vi "Draw Icon.vi"(6 "State":T2, 7 "Sizes":T1, 11 "Picture  In":picture) -> (3 "Picture":picture)   [LabVIEW 2020, in "FlexBlock.xnode"]
uses:
  FlexBlock.xnode
  State.ctl
  FlexBlocks/Type Descriptor.ctl
  FlexBlocks/Terminal Direction.ctl
  FlexBlocks/Value Mode.ctl
  FlexBlocks/Terminal State.ctl
  FlexBlocks/Special Terminal.ctl
  FlexBlocks/Errors.ctl
  <vilib>/picture/picture.llb/imagedata.ctl
  FlexBlocks/Calculated Sizes.ctl
  FlexBlocks/Size Constants.ctl
  FlexBlocks/FlexBlocks.lvlib
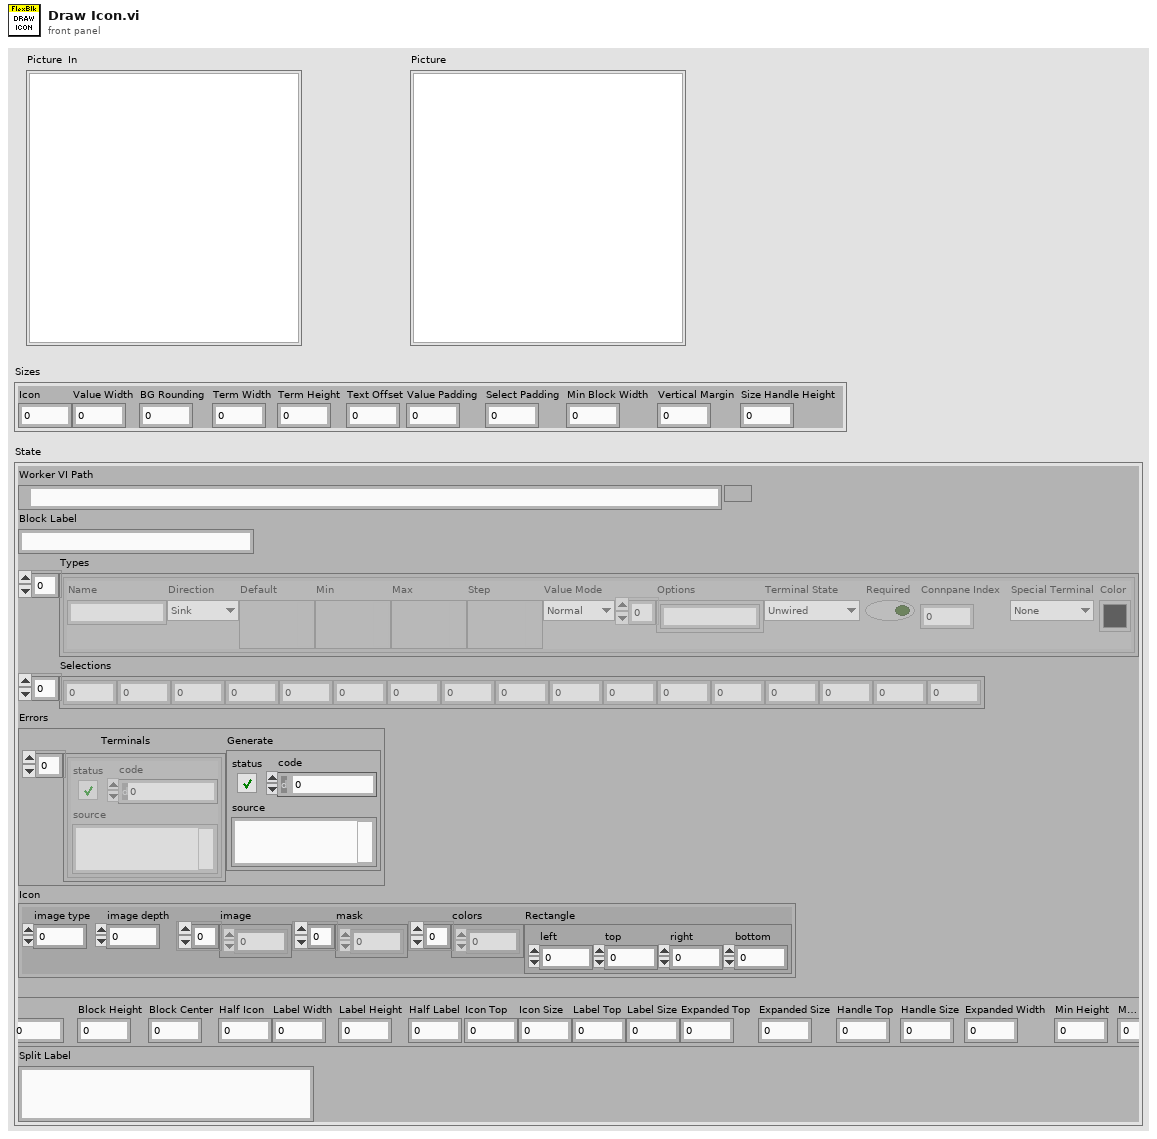
[diagram p1: front panel]
types:
  T1 = typedef "FlexBlocks.lvlib/Size Constants.ctl" = cluster{"Icon":i32, "Value Width":i32, "BG Rounding":i32, "Term Width":i32, "Term Height":i32, "Text Offset":i32, "Value Padding":i32, "Select Padding":i32, "Min Block Width":i32, "Vertical Margin":i32, "Size Handle Height":i32}
  T2 = typedef "FlexBlock.xnode/State.ctl" = cluster{"Worker VI Path":path, "Block Label":string, "Types":T3[], "Selections":i32[], "Errors":T8, "Icon":T9, "Calcd Sizes":T10, "Split Label":string}
  T3 = typedef "FlexBlocks.lvlib/Type Descriptor.ctl" = cluster{"Name":string, "Direction":T4, "Default":variant, "Min":variant, "Max":variant, "Step":variant, "Value Mode":T5, "Options":string[], "Terminal State":T6, "Required":bool, "Connpane Index":i32, "Special Terminal":T7, "Color":u32}
  T4 = typedef "FlexBlocks.lvlib/Terminal Direction.ctl" = enum16{"Sink", "Source"}
  T5 = typedef "FlexBlocks.lvlib/Value Mode.ctl" = enum16{"Normal", "Range", "Select"}
  T6 = typedef "FlexBlocks.lvlib/Terminal State.ctl" = enum16{"Unwired", "BadType", "BadRef", "Channel", "Value", "Control Ref"}
  T7 = typedef "FlexBlocks.lvlib/Special Terminal.ctl" = enum16{"None", "Action", "Init", "Tag", "State in", "State out", "Error"}
  T8 = typedef "FlexBlocks.lvlib/Errors.ctl" = cluster{"Terminals":errorcluster[], "Generate":errorcluster}
  T9 = typedef "imagedata.ctl" = cluster{"image type":i32, "image depth":i32, "image":u8[], "mask":u8[], "colors":u32[], "Rectangle":cluster{"left":i16, "top":i16, "right":i16, "bottom":i16}}
  T10 = typedef "FlexBlocks.lvlib/Calculated Sizes.ctl" = cluster{"Text Width":i32, "Text Height":i32, "Half Text":i32, "Block Width":i32, "Block Height":i32, "Block Center":i32, "Half Icon":i32, "Label Width":i32, "Label Height":i32, "Half Label":i32, "Icon Top":i32, "Icon Size":i32, "Label Top":i32, "Label Size":i32, "Expanded Top":i32, "Expanded Size":i32, "Handle Top":i32, "Handle Size":i32, "Expanded Width":i32, "Min Height":i32, "Max Height":i32}
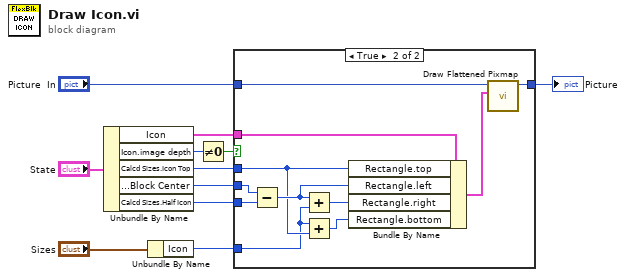
[diagram p0: block diagram]
diagram:
  n1 = Unbundle By Name("State") -> ("Icon"=w5:T9, "Icon.image depth"=w9:i32, "Calcd Sizes.Icon Top"=w4:i32, "Calcd Sizes.Block Center"=w3:i32, "Calcd Sizes.Half Icon"=w1:i32)
  n2 = Unbundle By Name("Sizes") -> ("Icon"=w2:i32)
  n3 = Not Equal To 0?(x=w9) -> (x != 0?=w6:bool)
  n4 = case shown="True" w6 {
    tunnel: "Picture  In" -> [w12 w23]
    tunnel: [w12 w22] -> w7
    tunnel: w5 -> [_ w21]
    tunnel: w4 -> [_ w15]
    tunnel: w3 -> [_ w20]
    tunnel: w2 -> [_ w14]
    tunnel: w1 -> [_ w19]
    frame False {
    }
    frame True {
      n5 = Subtract(x=w20, y=w19) -> (x-y=w18:i32)
      n6 = Add(x=w18, y=w14) -> (x+y=w17:i32)
      n7 = Add(x=w14, y=w15) -> (x+y=w16:i32)
      n8 = Bundle By Name(cluster=w21, "Rectangle.top"=w15, "Rectangle.left"=w18, "Rectangle.right"=w17, "Rectangle.bottom"=w16) -> (w13:T9)
      n9 = call <vilib>:"Draw Flattened Pixmap.vi"("image data"=w13, "picture"=w23) -> ("new picture"=w22:picture)  [unwired: 7 in]
    }
  }
  "Picture" <- w7
